vi "Read Tektronix WFM dimention.vi"(8 "Error In":errorcluster, 10 "offset (in bytes) (0)":i64, 11 "WFM file ref":T1={"refnum"=refnum, "byte order"=enum."little-endian", "Version"=0}) -> (0 "Error Out":errorcluster, 2 "Dimension":T2, 3 "WFM file ref out":T1={"refnum"=refnum, "byte order"=enum."little-endian", "Version"=0})   [LabVIEW 2015]
uses:
  WFM exp dimension.ctl
  WFM file ref.ctl
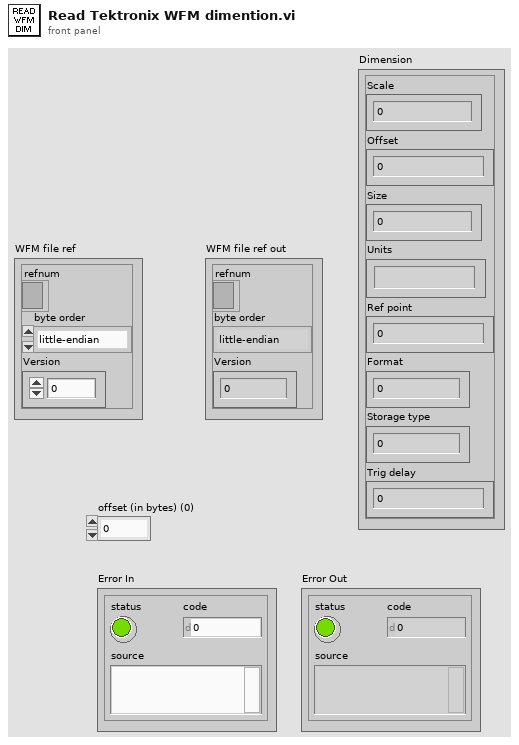
[diagram p1: front panel]
types:
  T1 = typedef "WFM file ref.ctl" = cluster{"refnum":refnum<file>, "byte order":enum16{"big-endian, network order", "native, host order", "little-endian"}, "Version":i32}
  T2 = typedef "WFM exp dimension.ctl" = cluster{"Scale":dbl, "Offset":dbl, "Size":i32, "Units":string, "Ref point":dbl, "Format":i32, "Storage type":i32, "Trig delay":dbl}
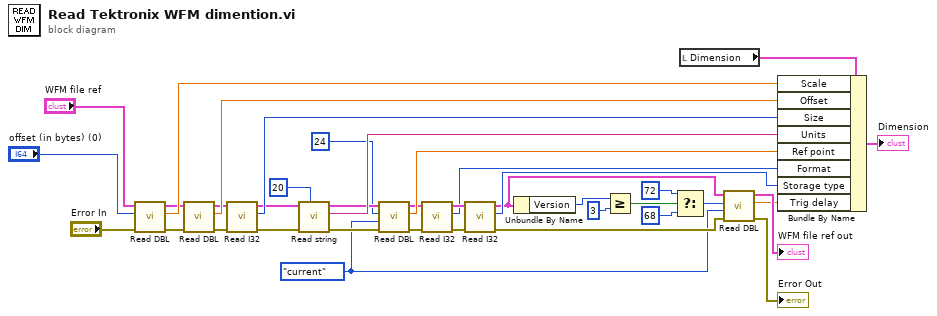
[diagram p0: block diagram]
diagram:
  w1 = enum16{"start", "end", "current"}."current" ("from (0:start)")
  n1 = call "Read DBL.vi"("Error In"="Error In", "offset (in bytes) (0)"="offset (in bytes) (0)", "WFM file ref"="WFM file ref") -> ("Error Out"=w36:errorcluster, "data"=w37:dbl, "WFM file ref out"=w35:T1)  [unwired: 6 in]
  n2 = call "Read DBL.vi"("Error In"=w36, "WFM file ref"=w35) -> ("Error Out"=w32:errorcluster, "data"=w34:dbl, "WFM file ref out"=w33:T1)  [unwired: 7 in]
  n3 = call "Read I32.vi"("Error In"=w32, "WFM file ref"=w33) -> ("Error Out"=w30:errorcluster, "data"=w31:i32, "WFM file ref out"=w29:T1)  [unwired: 7 in]
  n4 = call "Read string.vi"("count (1)"=20, "Error In"=w30, "WFM file ref"=w29) -> ("Error Out"=w24:errorcluster, "data"=w27:string, "WFM file ref out"=w25:T1)  [unwired: 6 in]
  n5 = call "Read DBL.vi"("Error In"=w24, "from (0:start)"=w1, "offset (in bytes) (0)"=i64 24, "WFM file ref"=w25) -> ("Error Out"=w20:errorcluster, "data"=w23:dbl, "WFM file ref out"=w22:T1)  [unwired: 5 in]
  n6 = call "Read I32.vi"("Error In"=w20, "WFM file ref"=w22) -> ("Error Out"=w19:errorcluster, "data"=w17:i32, "WFM file ref out"=w21:T1)  [unwired: 7 in]
  n7 = call "Read I32.vi"("Error In"=w19, "WFM file ref"=w21) -> ("Error Out"=w12:errorcluster, "data"=w18:i32, "WFM file ref out"=w9:T1)  [unwired: 7 in]
  n8 = Unbundle By Name(w9) -> ("Version"=w8:i32)
  n9 = Greater Or Equal?(x=w8, y=3) -> (x >= y?=w6:bool)
  n10 = Select(t=i64 72, s=w6, f=i64 68) -> (s? t:f=w3:i64)
  n11 = local read "Dimension"() -> (w15:T2)
  n12 = call "Read DBL.vi"("Error In"=w12, "from (0:start)"=w1, "offset (in bytes) (0)"=w3, "WFM file ref"=w9) -> ("Error Out"=→"Error Out":errorcluster, "data"=w10:dbl, "WFM file ref out"=→"WFM file ref out":T1)  [unwired: 5 in]
  n13 = Bundle By Name(cluster=w15, "Scale"=w37, "Offset"=w34, "Size"=w31, "Units"=w27, "Ref point"=w23, "Format"=w17, "Storage type"=w18, "Trig delay"=w10) -> (→"Dimension":T2)
